vi "Test Configuration Panel Template.vi"(6 "Write? (f)":bool, 7 "Connection Refnum":T2, 8 "error in (no error)":errorcluster, 9 "Configuration (\"\")":string, 11 "Template Keys (empty)":T1) -> (0 "error out":errorcluster, 1 "Configuration":string, 3 "Template Keys":T1, 5 "Connection Refnum":T2)   [LabVIEW 2011]
uses:
  Summitek/Win32/ODBC/SQL Controls/Connection Refnum.ctl
  ITK/utils/keyedarr.llb/Keyed Array.ctl
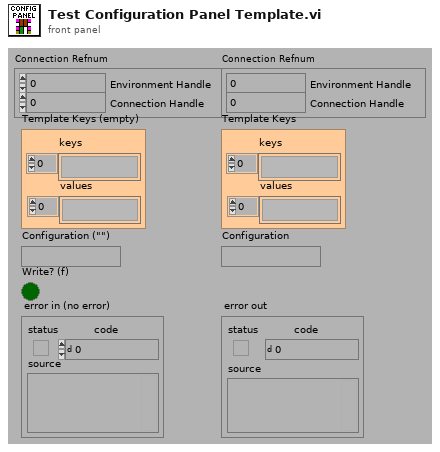
[diagram p1: front panel]
types:
  T1 = typedef "Keyed Array.ctl" = cluster{"keys":string[], "values":string[]}
  T2 = typedef "Connection Refnum.ctl" = cluster{"Environment Handle":i32, "Connection Handle":i32}
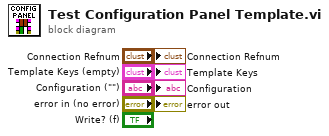
[diagram p0: block diagram]
diagram:
